vi "GPS.vi"() -> ()   [LabVIEW 2020]
uses:
  <vilib>/Instr/_visa.llb/VISA Configure Serial Port (Instr).vi
panel:
  in  "Tab Control":enum32{"Parsing Data", "Graph(Present)"}(tab)
  out "GNVTG":string[](array[string])
  out "GNRMC":string[](array[string])
  out "GNGGA":string[](array[string])
  in  "stop":bool
  in  "VISA resource name":refnum<visa-resource-name>
  in  "baud rate (115200)":u32=9600
  out "True Heading":string
  out "time":dbl
  out "Longtitude":dbl
  out "Latitude":dbl
  out "error out":errorcluster
  out "도 2":string
  out "도분초(lat)":string
  out "Y(E)":dbl format="%#_6f"
  out "X(N)":dbl format="%#_6f"
  out "도":string
  out "도분초(lon)":string
  out "XY Graph":cluster{"array":dbl[], "array":dbl[]}[](graph)
  out "x .and. y?":bool
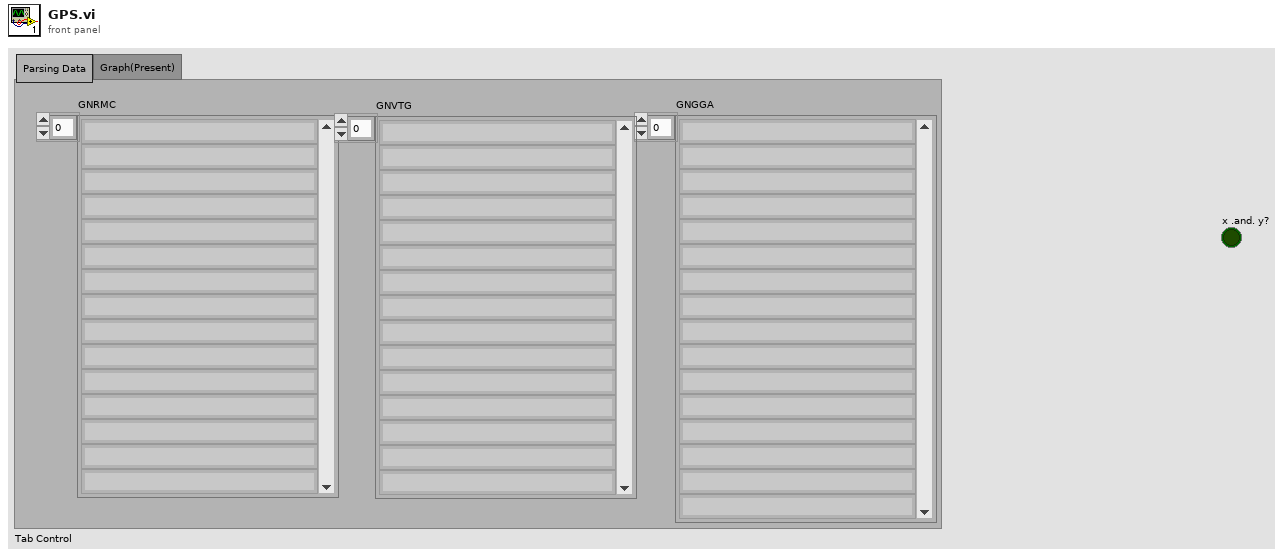
[diagram p1: front panel]
types:
  T1 = enum16{"open", "replace", "create", "open or create", "replace or create", "replace or create with confirmation"}
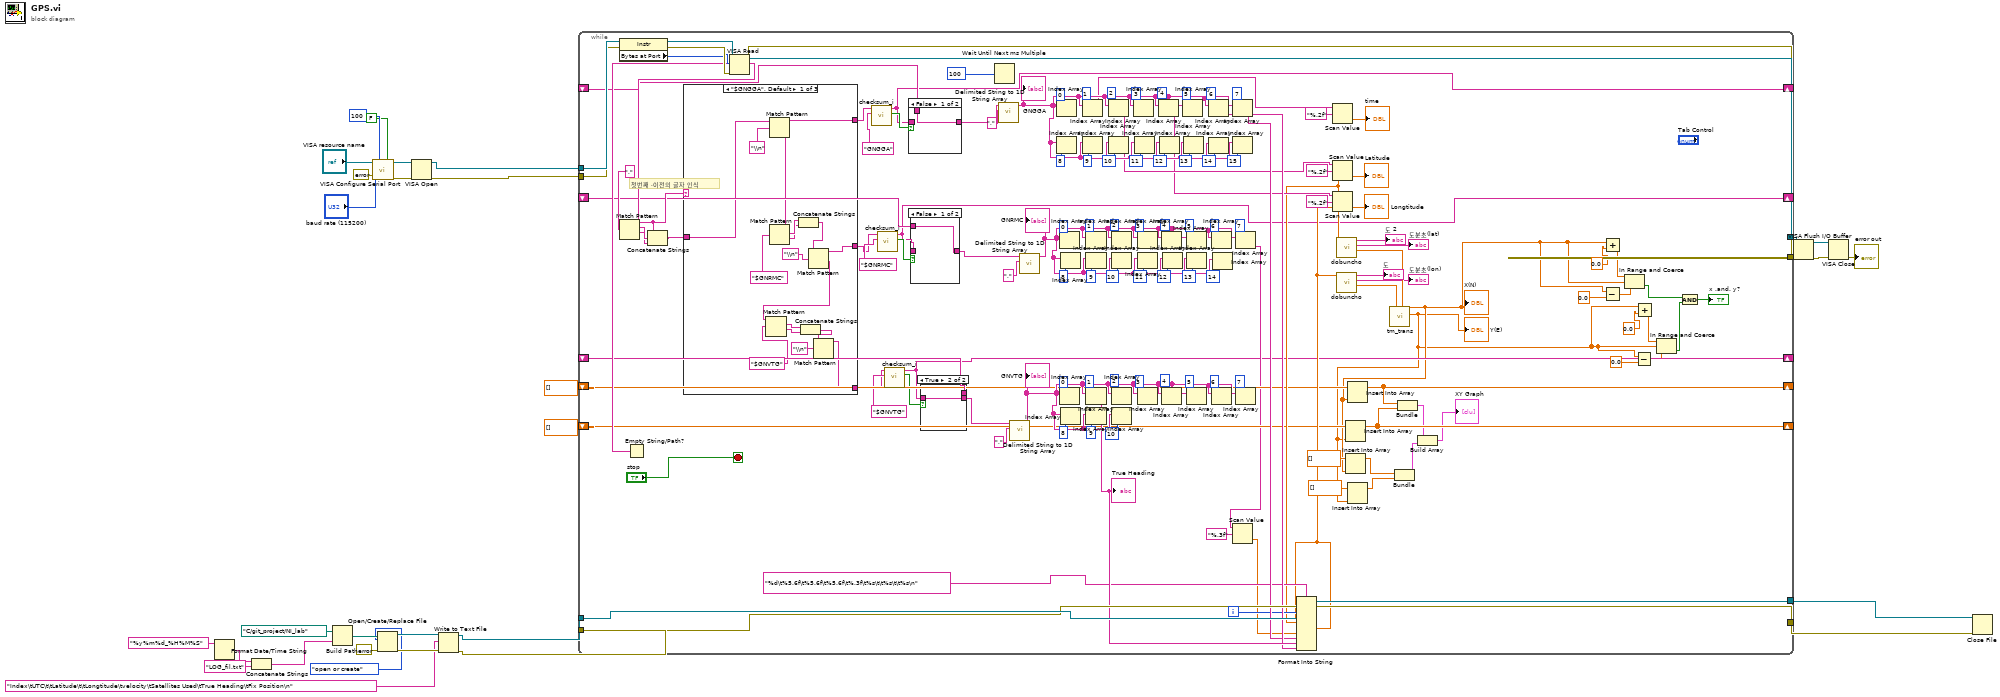
[diagram p0: block diagram]
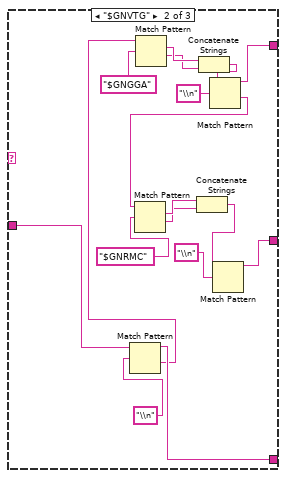
[diagram p5: hidden frame]
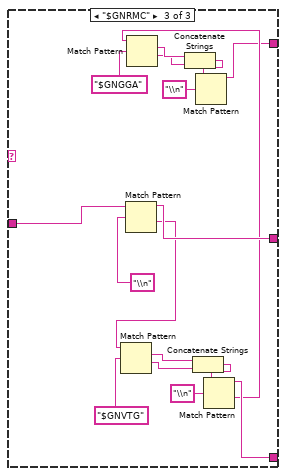
[diagram p6: hidden frame]
diagram:
  n1 = Format Date/Time String(time format string (%c)="%y%m%d_%H%M%S") -> (date/time string=w3:string)  [unwired: 2 in]
  n2 = Concatenate Strings(w3, "LOG_fil.txt" ("string")) -> (w1:string)
  n3 = Build Path(base path=path "C:/git_project/NI_lab", name or relative path=w1) -> (appended path=w29:path)
  n4 = call-poly "VISA Configure Serial Port"("VISA resource name"="VISA resource name", "timeout (10sec)"=u32 100, "Enable Termination\nChar (T)"=FALSE ("Enable Termination\nChar (T)"), "baud rate (9600)"="baud rate (115200)", "error in (no error)"=errorcluster {"status"=FALSE, "code"=0, "source"=""}) -> ("VISA resource name out"=w15:refnum<visa-resource-name>, "error out"=w16:errorcluster)  [unwired: 9 in]
  n5 = Open/Create/Replace File(file path (use dialog)=w29, error in=errorcluster {"status"=FALSE, "code"=0, "source"=""}, operation (0:open)=T1."open or create") -> (refnum out=w30:refnum<file>, error out=w31:errorcluster)  [unwired: 3 in, 1 out]
  n6 = VISA Open(error in (no error)=w16, VISA resource name=w15) -> (VISA resource name=w14:refnum<visa-resource-name>, error out=w13:errorcluster)  [unwired: 3 in]
  n7 = Write to Text File(file (use dialog)=w30, text="Index\tUTC\t\tLatitude\t\tLongtitude\tvelocity\tSatellites Used\tTrue Heading\tFix Position\n", error in=w31) -> (refnum out=w22:refnum<file>, error out=w21:errorcluster)  [unwired: 1 in, 1 out]
  n8 = while {
    tunnel: w21 -> [w113]
    tunnel: [w112] -> w23
    tunnel: w22 -> [w115]
    tunnel: [w114] -> w24
    tunnel: w14 -> [w110]
    tunnel: w13 -> [w109]
    tunnel: [w98] -> w12
    tunnel: [w97] -> w11
    shift-right: [w54] -> _
    shift-left: _ -> [w76]
    shift-right: [w50] -> _
    shift-left: _ -> [w74]
    shift-right: [w47] -> _
    shift-left: _ -> [w72]
    shift-right: [w70] -> _
    shift-left: dbl[] [] -> [w71]
    shift-right: [w68] -> _
    shift-left: dbl[] [] -> [w69]
    i -> [w96]
    stop <- "stop" stop-if-true
    # "첫번째 ,이전의 글자 인식"
    n9 = property class="Instr"(reference=w110, error in=w109) -> (reference out=w108:refnum<visa-resource-name>, error out=w107:errorcluster, "Bytes at Port"=w95:u32)
    n10 = VISA Read(VISA resource name=w108, byte count=w95, error in (no error)=w107) -> (VISA resource name out=w98:refnum<visa-resource-name>, read buffer=w89:string, error out=w97:errorcluster)  [unwired: 1 out]
    n11 = Match Pattern(string=w89, regular expression=",") -> (before substring=w86:string, match substring=w85:string, after substring=w84:string)  [unwired: 1 in, 1 out]
    n12 = Empty String/Path?(string/path=w89) -> ()  [unwired: 1 out]
    n13 = Concatenate Strings(w86, w85, w84) -> (w87:string)
    n14 = case shown="\"$GNGGA\", Default" w86 {
      tunnel: w87 -> [w185 w202 w217]
      tunnel: [w184 w194 w204] -> w56
      tunnel: [w177 w187 w216] -> w52
      tunnel: [w170 w200 w210] -> w48
      frame "$GNGGA", Default {
        n15 = Match Pattern(string=w185, regular expression="\\n") -> (before substring=w184:string, after substring=w183:string)  [unwired: 1 in, 2 out]
        n16 = Match Pattern(string=w183, regular expression="$GNRMC") -> (match substring=w180:string, after substring=w179:string)  [unwired: 1 in, 2 out]
        n17 = Concatenate Strings(w180, w179) -> (w178:string)
        n18 = Match Pattern(string=w178, regular expression="\\n") -> (before substring=w177:string, after substring=w174:string)  [unwired: 1 in, 2 out]
        n19 = Match Pattern(string=w174, regular expression="$GNVTG") -> (match substring=w172:string, after substring=w171:string)  [unwired: 1 in, 2 out]
        n20 = Concatenate Strings(w172, w171) -> (w175:string)
        n21 = Match Pattern(string=w175, regular expression="\\n") -> (before substring=w170:string)  [unwired: 1 in, 3 out]
      }
      frame "$GNVTG" {
        n22 = Match Pattern(string=w202, regular expression="\\n") -> (before substring=w200:string, after substring=w199:string)  [unwired: 1 in, 2 out]
        n23 = Match Pattern(string=w199, regular expression="$GNGGA") -> (match substring=w196:string, after substring=w195:string)  [unwired: 1 in, 2 out]
        n24 = Concatenate Strings(w196, w195) -> (w197:string)
        n25 = Match Pattern(string=w197, regular expression="\\n") -> (before substring=w194:string, after substring=w193:string)  [unwired: 1 in, 2 out]
        n26 = Match Pattern(string=w193, regular expression="$GNRMC") -> (match substring=w189:string, after substring=w188:string)  [unwired: 1 in, 2 out]
        n27 = Concatenate Strings(w189, w188) -> (w190:string)
        n28 = Match Pattern(string=w190, regular expression="\\n") -> (before substring=w187:string)  [unwired: 1 in, 3 out]
      }
      frame "$GNRMC" {
        n29 = Match Pattern(string=w217, regular expression="\\n") -> (before substring=w216:string, after substring=w215:string)  [unwired: 1 in, 2 out]
        n30 = Match Pattern(string=w215, regular expression="$GNVTG") -> (match substring=w211:string, after substring=w212:string)  [unwired: 1 in, 2 out]
        n31 = Concatenate Strings(w211, w212) -> (w213:string)
        n32 = Match Pattern(string=w213, regular expression="\\n") -> (before substring=w210:string, after substring=w209:string)  [unwired: 1 in, 2 out]
        n33 = Match Pattern(string=w209, regular expression="$GNGGA") -> (match substring=w206:string, after substring=w205:string)  [unwired: 1 in, 2 out]
        n34 = Concatenate Strings(w206, w205) -> (w207:string)
        n35 = Match Pattern(string=w207, regular expression="\\n") -> (before substring=w204:string)  [unwired: 1 in, 3 out]
      }
    }
    n36 = call "checksum_i.vi"("check dataName"="GNGGA", "string"=w56) -> ("Boolean"=w55:bool, "String"=w54:string)  [unwired: 8 in]
    n37 = call "checksum_i.vi"("check dataName"="$GNRMC", "string"=w52) -> ("Boolean"=w51:bool, "String"=w50:string)  [unwired: 8 in]
    n38 = call "checksum_i.vi"("check dataName"="$GNVTG", "string"=w48) -> ("Boolean"=w46:bool, "String"=w47:string)  [unwired: 8 in]
    n39 = case shown="False" w55 {
      tunnel: [w168 w169] -> w77
      tunnel: w54 -> [_ w169]
      tunnel: w76 -> [w168 _]
      frame False {
      }
      frame True {
      }
    }
    n40 = case shown="False" w51 {
      tunnel: w50 -> [_ w167]
      tunnel: [w166 w167] -> w75
      tunnel: w74 -> [w166 _]
      frame False {
      }
      frame True {
      }
    }
    n41 = case shown="True" w46 {
      tunnel: w47 -> [_ w165]
      tunnel: [w164 w165] -> w73
      tunnel: w72 -> [w164 _]
      frame False {
      }
      frame True {
      }
    }
    n42 = Wait Until Next ms Multiple(millisecond multiple=u32 100) -> ()  [unwired: 1 out]
    n43 = call <vilib>:"Delimited String to 1D String Array.vi"("delimiter"=",", "delimited string"=w77) -> ("string array"=w162:string[])  [unwired: 9 in]
    "GNGGA" <- w162
    n44 = call <vilib>:"Delimited String to 1D String Array.vi"("delimiter"=",", "delimited string"=w73) -> ("string array"=w127:string[])  [unwired: 9 in]
    "GNVTG" <- w127
    n45 = call <vilib>:"Delimited String to 1D String Array.vi"("delimiter"=",", "delimited string"=w75) -> ("string array"=w144:string[])  [unwired: 9 in]
    "GNRMC" <- w144
    n46 = Index Array(array=w162, index=0) -> ()  [unwired: 1 out]
    n47 = Index Array(array=w162, index=8) -> ()  [unwired: 1 out]
    n48 = Index Array(array=w144, index=0) -> ()  [unwired: 1 out]
    n49 = Index Array(array=w127, index=0) -> ()  [unwired: 1 out]
    n50 = Index Array(array=w144, index=8) -> ()  [unwired: 1 out]
    n51 = Index Array(array=w127, index=8) -> ()  [unwired: 1 out]
    n52 = Index Array(array=w162, index=1) -> (element=w103:string)
    n53 = Index Array(array=w162, index=9) -> ()  [unwired: 1 out]
    n54 = Index Array(array=w144, index=1) -> ()  [unwired: 1 out]
    n55 = Index Array(array=w144, index=9) -> ()  [unwired: 1 out]
    n56 = Index Array(array=w127, index=1) -> (element=w106:string)
    "True Heading" <- w106
    n57 = Index Array(array=w127, index=9) -> ()  [unwired: 1 out]
    n58 = Index Array(array=w162, index=2) -> (element=w100:string)
    n59 = Index Array(array=w162, index=10) -> ()  [unwired: 1 out]
    n60 = Index Array(array=w144, index=2) -> ()  [unwired: 1 out]
    n61 = Index Array(array=w144, index=10) -> ()  [unwired: 1 out]
    n62 = Index Array(array=w127, index=2) -> ()  [unwired: 1 out]
    n63 = Index Array(array=w127, index=10) -> ()  [unwired: 1 out]
    n64 = Index Array(array=w162, index=3) -> ()  [unwired: 1 out]
    n65 = Index Array(array=w162, index=11) -> ()  [unwired: 1 out]
    n66 = Index Array(array=w144, index=3) -> ()  [unwired: 1 out]
    n67 = Index Array(array=w127, index=3) -> ()  [unwired: 1 out]
    n68 = Index Array(array=w144, index=11) -> ()  [unwired: 1 out]
    n69 = Index Array(array=w162, index=4) -> (element=w99:string)
    n70 = Index Array(array=w162, index=12) -> ()  [unwired: 1 out]
    n71 = Index Array(array=w144, index=4) -> ()  [unwired: 1 out]
    n72 = Index Array(array=w127, index=4) -> ()  [unwired: 1 out]
    n73 = Index Array(array=w144, index=12) -> ()  [unwired: 1 out]
    n74 = Index Array(array=w162, index=5) -> ()  [unwired: 1 out]
    n75 = Index Array(array=w162, index=13) -> ()  [unwired: 1 out]
    n76 = Index Array(array=w144, index=5) -> ()  [unwired: 1 out]
    n77 = Index Array(array=w127, index=5) -> ()  [unwired: 1 out]
    n78 = Index Array(array=w144, index=13) -> ()  [unwired: 1 out]
    n79 = Index Array(array=w162, index=6) -> (element=w105:string)
    n80 = Index Array(array=w162, index=14) -> ()  [unwired: 1 out]
    n81 = Index Array(array=w144, index=6) -> ()  [unwired: 1 out]
    n82 = Index Array(array=w127, index=6) -> ()  [unwired: 1 out]
    n83 = Index Array(array=w144, index=14) -> ()  [unwired: 1 out]
    n84 = Index Array(array=w162, index=7) -> (element=w104:string)
    n85 = Index Array(array=w162, index=15) -> ()  [unwired: 1 out]
    n86 = Index Array(array=w144, index=7) -> (element=w60:string)
    n87 = Scan Value(string=w60, format string="%.3f") -> (value=w59:dbl)  [unwired: 1 in, 1 out]
    n88 = Index Array(array=w127, index=7) -> ()  [unwired: 1 out]
    n89 = Scan Value(string=w103, format string="%.2f") -> (value=→"time":dbl)  [unwired: 1 in, 1 out]
    n90 = Scan Value(string=w100, format string="%.2f") -> (value=w82:dbl)  [unwired: 1 in, 1 out]
    "Latitude" <- w82
    n91 = Scan Value(string=w99, format string="%.2f") -> (value=w81:dbl)  [unwired: 1 in, 1 out]
    "Longtitude" <- w81
    n92 = Format Into String(format string="%d\t%5.6f\t%5.6f\t%5.6f\t%.3f\t%s\t\t%s\t\t%s\n", initial string=w115, error in=w113, w96, w81, w82, w81, w59, w104, w106, w105) -> (resulting string=w114:refnum<file>, error out=w112:errorcluster)
    n93 = call "dobuncho.vi"("Numeric in"=w82) -> ("Numeric out"=w83:dbl, "String"=→"도분초(lat)":string, "String 2"=→"도 2":string)  [unwired: 8 in]
    n94 = call "dobuncho.vi"("Numeric in"=w81) -> ("Numeric out"=w78:dbl, "String"=→"도분초(lon)":string, "String 2"=→"도":string)  [unwired: 8 in]
    n95 = call "tm_trans.vi"("Long"=w78, "Lat"=w83) -> ("Numeric"=w33:dbl, "out_pt"=w34:dbl)  [unwired: 8 in]
    "Y(E)" <- w33
    "X(N)" <- w34
    n96 = Insert Into Array(array=w69, new element=w33) -> (w68:dbl[])  [unwired: 1 in]
    n97 = Insert Into Array(array=dbl[] [], new element=w34) -> (w65:dbl[])  [unwired: 1 in]
    n98 = Insert Into Array(array=dbl[] [], new element=w33) -> (w64:dbl[])  [unwired: 1 in]
    n99 = Insert Into Array(array=w71, new element=w34) -> (w70:dbl[])  [unwired: 1 in]
    n100 = Bundle("array"=w65, "array"=w64) -> (w63:cluster{"array":dbl[], "array":dbl[]})  [unwired: 1 in]
    n101 = Bundle(w70, w68) -> (w62:cluster{dbl[], dbl[]})  [unwired: 1 in]
    n102 = Build Array(w62, w63) -> (→"XY Graph":cluster{"array":dbl[], "array":dbl[]}[])
    n103 = Subtract(x=w34, y=0.0 ("lower limit")) -> (x-y=w42:dbl)
    n104 = Add(x=w34, y=0.0 ("upper limit")) -> (x+y=w44:dbl)
    n105 = In Range and Coerce(upper limit=w44, x=w34, lower limit=w42) -> (In Range?=w36:bool)  [unwired: 1 out]
    n106 = Subtract(x=w33, y=0.0 ("lower limit")) -> (x-y=w38:dbl)
    n107 = Add(x=w33, y=0.0 ("upper limit")) -> (x+y=w40:dbl)
    n108 = In Range and Coerce(upper limit=w40, x=w33, lower limit=w38) -> (In Range?=w37:bool)  [unwired: 1 out]
    n109 = And(x=w36, y=w37) -> (x .and. y?=→"x .and. y?":bool)
  }
  n110 = VISA Flush I/O Buffer(VISA resource name=w12, error in (no error)=w11) -> (VISA resource name out=w9:refnum<visa-resource-name>, error out=w10:errorcluster)  [unwired: 1 in]
  n111 = VISA Close(VISA resource name=w9, error in (no error)=w10) -> (error out=→"error out":errorcluster)
  n112 = Close File(refnum=w24, error in=w23) -> ()  [unwired: 2 out]
